vi "Commit to Include File.vi"(8 "error in (no error)":errorcluster, 11 "Coverage Report in":refnum<class "Coverage Report.lvclass">) -> (0 "error out":errorcluster, 3 "Coverage Report out":refnum<class "Coverage Report.lvclass">)   [LabVIEW 2020, in "Coverage Report.lvclass"]
uses:
  Coverage Report.lvclass
  Coverage Report.lvclass/Coverage Report.ctl
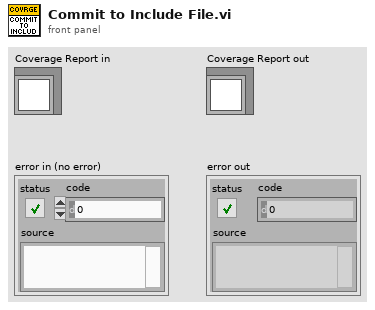
[diagram p1: front panel]
types:
  T1 = enum16{"open", "replace", "create", "open or create", "replace or create", "replace or create with confirmation"}
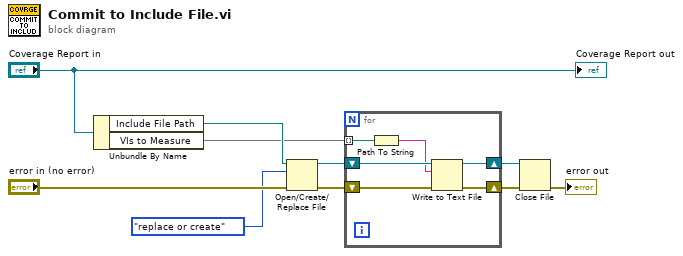
[diagram p0: block diagram]
diagram:
  n1 = Unbundle By Name("Coverage Report in") -> ("Include File Path"=w7:path, "VIs to Measure"=w1:set{path})
  n2 = Open/Create/Replace File(file path (use dialog)=w7, error in="error in (no error)", operation (0:open)=T1."replace or create") -> (refnum out=w4:refnum<file>, error out=w8:errorcluster)  [unwired: 3 in, 1 out]
  n3 = for {
    shift-right: [w15] -> w5
    shift-left: w8 -> [w16]
    shift-right: [w13] -> w2
    shift-left: w4 -> [w14]
    tunnel: w1 -> [w12] mode=indexing
    n4 = Path To String(path=w12) -> (string=w11:string)
    n5 = Write to Text File(file (use dialog)=w14, text=w11, error in=w16) -> (refnum out=w13:refnum<file>, error out=w15:errorcluster)  [unwired: 1 in, 1 out]
  }
  n6 = Close File(refnum=w2, error in=w5) -> (error out=→"error out":errorcluster)  [unwired: 1 out]
  "Coverage Report out" <- "Coverage Report in"
